vi "log time since last call to file.vi"(0 "Position Identifier (for log messages)":string, 11 "error in (no error)":errorcluster caption="error in") -> (15 "error out":errorcluster)   [LabVIEW 2012]
uses:
  resource/Public/Subs/ViServer/Message Logger Fuction.ctl
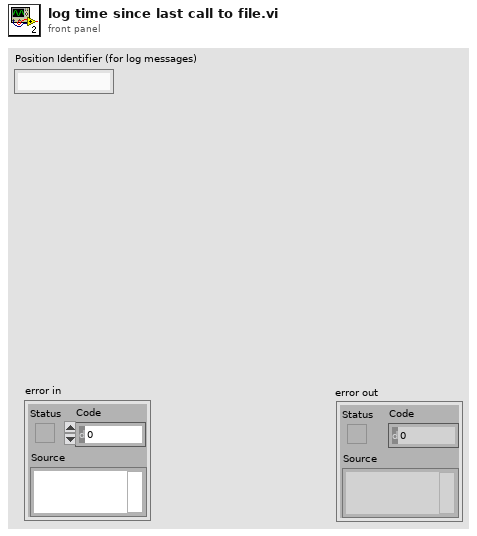
[diagram p1: front panel]
types:
  T1 = typedef "Message Logger Fuction.ctl" = enum16{"set config", "log messages", "log errors", "log & del err"}
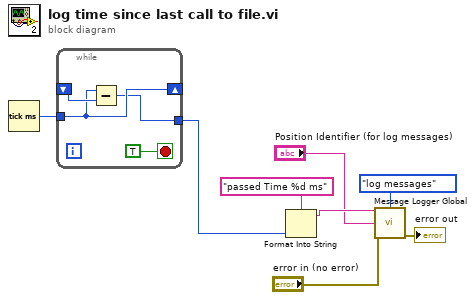
[diagram p0: block diagram]
diagram:
  n1 = Tick Count (ms)() -> (millisecond timer value=w8:u32)
  n2 = while {
    tunnel: w8 -> [w11]
    shift-right: [w11] -> _
    shift-left: _ -> [w12]
    tunnel: [w10] -> w1
    stop <- TRUE stop-if-true
    n3 = Subtract(x=w11, y=w12) -> (x-y=w10:u32)
  }
  n4 = Format Into String(format string="passed Time %d ms", w1) -> (resulting string=w6:string)  [unwired: 2 in, 1 out]
  n5 = call "Message Logger Global.vi"("Message in"=w6, "Message Logger Function"=Message_Logger_Fuction."log messages", "Position Identifier (for log messages)"="Position Identifier (for log messages)", "error in (no error)"="error in (no error)") -> ("error out"=→"error out":errorcluster)  [unwired: 11 in]
